vi "Update Transaction with Category.vi"(8 "error in (no error)":errorcluster, 9 "Transaction":refnum<class "Transaction.lvclass">, 10 "Category ID":string, 11 "Database in":refnum<class "Database.lvclass">) -> (0 "error out":errorcluster, 3 "Database out":refnum<class "Database.lvclass">)   [LabVIEW 2018, in "Database.lvclass"]
uses:
  Database.lvclass
  Transaction/Transaction.lvclass
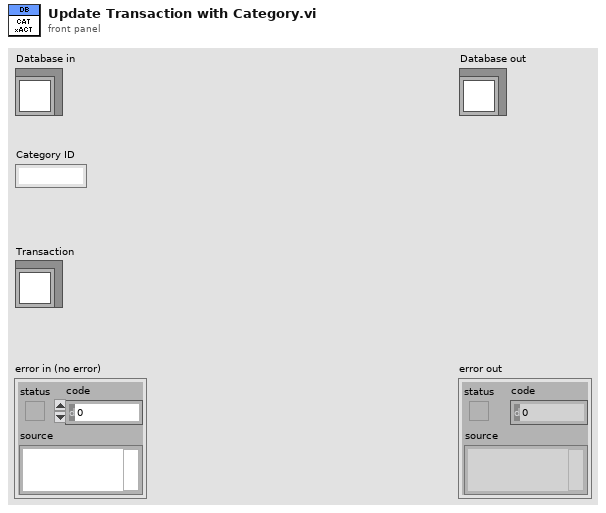
[diagram p1: front panel]
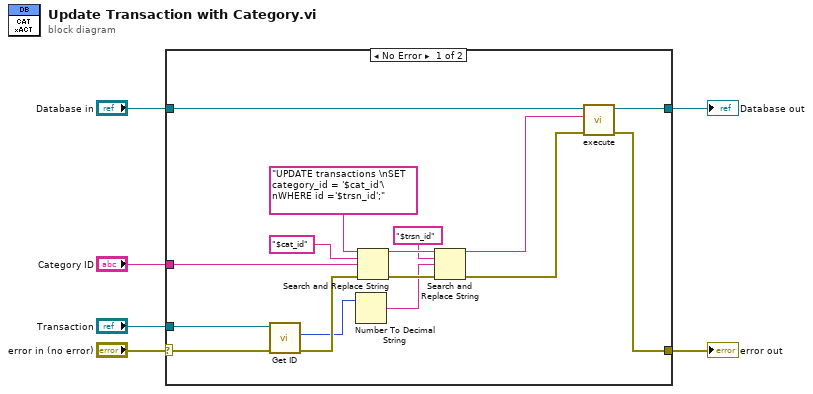
[diagram p0: block diagram]
diagram:
  n1 = case shown="No Error" "error in (no error)" {
    selector: "error in (no error)" -> [w9 w24]
    tunnel: [w20 w24] -> w5
    tunnel: [w22 w23] -> w3
    tunnel: "Database in" -> [w21 w23]
    tunnel: "Category ID" -> [w14 _]
    tunnel: "Transaction" -> [w11 _]
    frame No Error {
      n2 = call "Get ID.vi"("error in (no error)"=w9, "Transaction in"=w11) -> ("error out"=w8:errorcluster, "ID"=w7:i32)  [unwired: 7 in, 1 out]
      n3 = Number To Decimal String(number=w7) -> (decimal integer string=w10:string)  [unwired: 1 in]
      n4 = Search and Replace String(input string="UPDATE transactions \nSET category_id = '$cat_id'\nWHERE id ='$trsn_id';", search string="$cat_id", replace string=w14, error in=w8) -> (result string=w15:string, error out=w19:errorcluster)  [unwired: 4 in, 2 out]
      n5 = Search and Replace String(input string=w15, search string="$trsn_id", replace string=w10, error in=w19) -> (result string=w17:string, error out=w18:errorcluster)  [unwired: 4 in, 2 out]
      n6 = call "execute.vi"("error in (no error)"=w18, "SQL query"=w17, "Database in"=w21) -> ("error out"=w20:errorcluster, "Database out"=w22:refnum<class "Database.lvclass">)  [unwired: 7 in]
    }
    frame Error {
    }
  }
  "error out" <- w5
  "Database out" <- w3
